vi "flyback graph.vi"(6 "x pts flyback":i32, 9 "x pixels":i32, 10 "x max":dbl, 11 "x min":dbl) -> (3 "Array":dbl[](array[numeric]))   [LabVIEW 2012]
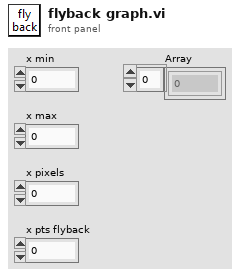
[diagram p1: front panel]
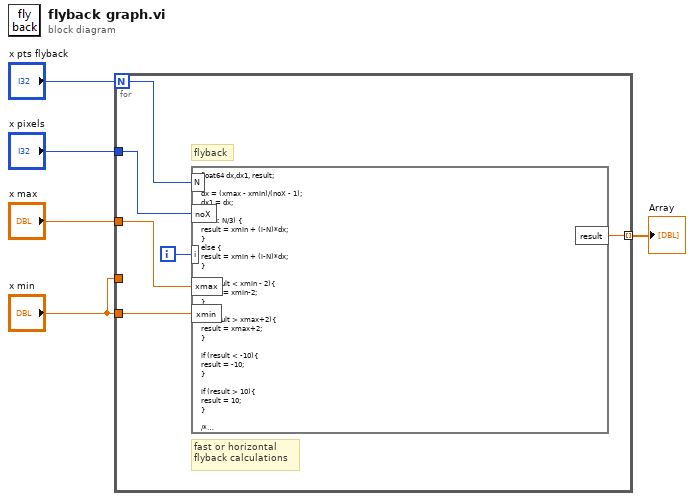
[diagram p0: block diagram]
diagram:
  n1 = for {
    N: "x pts flyback" -> [w11]
    tunnel: [w6] -> w5 mode=indexing
    tunnel: "x min" -> [_]
    tunnel: "x min" -> [w9]
    tunnel: "x max" -> [w8]
    tunnel: "x pixels" -> [w7]
    i -> [w10]
    # "flyback"
    # "fast or horizontal \nflyback calculations"
    n2 = formula code="float64 dx,dx1, result;\n\ndx = (xmax - xmin)/(noX - 1);\ndx1 = dx;\n\nif (i < N/3) {\nresult = xmin + (i-N)*dx; \n}\nelse {\nresult = xmin + (i-N)*dx;\n}\n\nif (result < xmin - 2){\nresult = xmin-2;\n}\n\nif (result > xmax+2){\nresult = xmax+2;\n}\n\nif (result < -10){\nresult = -10;\n}\n\nif (result > 10){\nresult = 10;\n}\n\n/*\nif (i < N/3) {\nresult = xmax + i*dx;\n}\nelse if (i< 2*N/3 & i >= N/3){\nresult = xmin;\n}\nelse {\nresult = xmin + i*dx - N*dx;\n}*/"("i"=w10, "N"=w11, "xmax"=w8, "xmin"=w9, "noX"=w7) -> ("result"=w6:dbl)
  }
  "Array" <- w5
